vi "conector2corriente.vi"(0 "salida":string[](array[string]), 1 "Salida ent":string, 2 "corriente entrada":dbl, 3 "polarizador":dbl[](array[numeric]), 4 "Polarizadorent":dbl, 5 "voltaje":dbl[](array[numeric]), 7 "VoltajeEnt":dbl, 10 "Enum":T1(ring), 11 "Indice":i32) -> (13 "VoltajeEnt 2":dbl, 14 "salida 2":string[](array[string]), 15 "Salida ent 2":string, 16 "corriente salida":dbl, 17 "polarizador 2":dbl[](array[numeric]), 18 "Polarizador":dbl, 19 "voltaje 2":dbl[](array[numeric]))   [LabVIEW 2016]
doc: "Este subVI selecciona al arreglo del cual se obtienen los valores que se enviarán a los dispositivos. \nLas entradas son tres arreglos y tres valores y de igual forma son las salidas."
panel:
  in  "corrientes":dbl[](array[numeric])
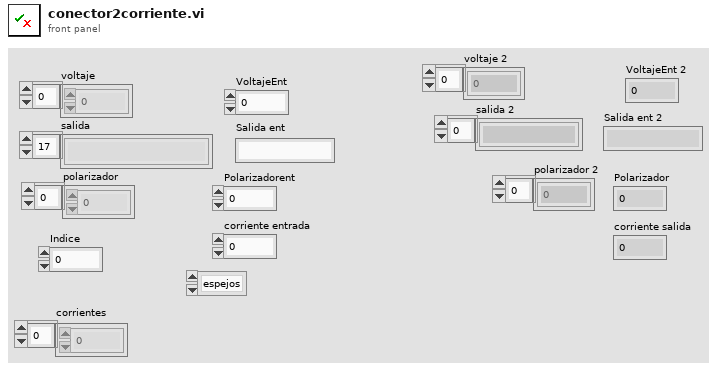
[diagram p1: front panel]
types:
  T1 = enum16{"espejos", "polarizador", "voltaje", "potenciometro ", "CCD", "lockin", "laser", "ninguno"}
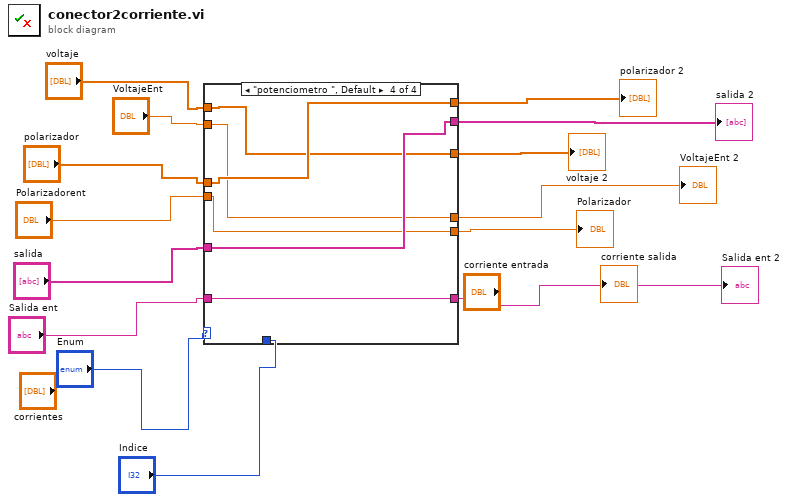
[diagram p0: block diagram]
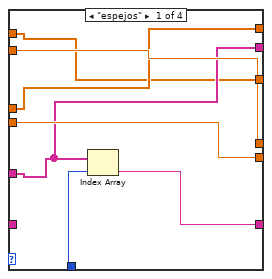
[diagram p2: hidden frame]
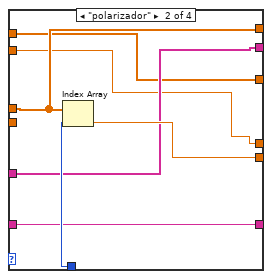
[diagram p3: hidden frame]
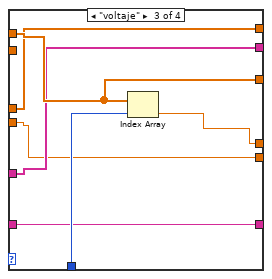
[diagram p4: hidden frame]
diagram:
  n1 = case shown="\"potenciometro \", Default" "Enum" {
    tunnel: "polarizador" -> [w20 w26 w29 w41]
    tunnel: "Indice" -> [w15 w28 w35 _]
    tunnel: [w19 w27 w30 w37] -> w12
    tunnel: [w20 w26 w29 w41] -> w11
    tunnel: "Polarizadorent" -> [w19 _ w30 w37]
    tunnel: "salida" -> [w17 w25 w32 w40]
    tunnel: "Salida ent" -> [_ w24 w31 w36]
    tunnel: "VoltajeEnt" -> [w21 w23 _ w38]
    tunnel: [w21 w23 w34 w38] -> w6
    tunnel: [w18 w24 w31 w36] -> w5
    tunnel: [w17 w25 w32 w40] -> w4
    tunnel: "voltaje" -> [w16 w22 w33 w39]
    tunnel: [w16 w22 w33 w39] -> w2
    frame "espejos" {
      n2 = Index Array(array=w17, index=w15) -> (element=w18:string)
    }
    frame "polarizador" {
      n3 = Index Array(array=w26, index=w28) -> (element=w27:dbl)
    }
    frame "voltaje" {
      n4 = Index Array(array=w33, index=w35) -> (element=w34:dbl)
    }
    frame "potenciometro ", Default {
    }
  }
  "Polarizador" <- w12
  "polarizador 2" <- w11
  "VoltajeEnt 2" <- w6
  "Salida ent 2" <- w5
  "salida 2" <- w4
  "voltaje 2" <- w2
